vi "servo new.vi"() -> ()   [LabVIEW 2017]
panel:
  in  "Duty Cycle (%)":dbl=50.0
  out "error out":errorcluster
  in  "error in (no error)":errorcluster
  in  "Phase":dbl
  in  "Amplitude":dbl=1.0
  in  "Frequency":dbl=10.0
  in  "Reset Signal":bool
  in  "Offset":dbl
  out "Waveform Graph":dynamicdata(graph)
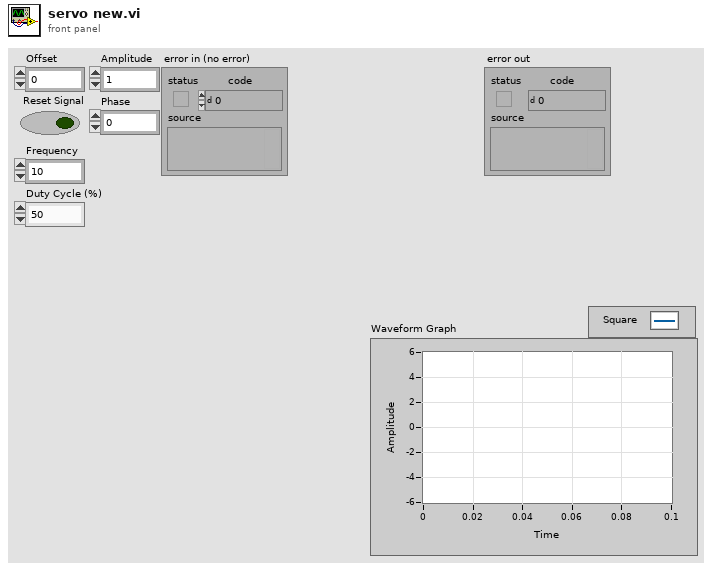
[diagram p1: front panel]
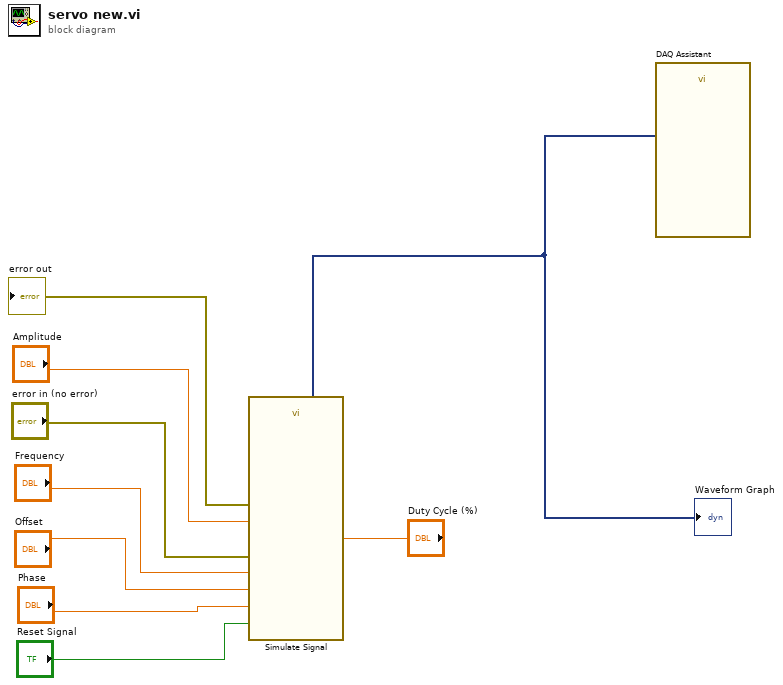
[diagram p0: block diagram]
diagram:
  n1 = call "Simulate Signal"("Offset"="Offset", "Duty Cycle (%)"="Duty Cycle (%)", "Reset Signal"="Reset Signal", "Frequency"="Frequency", "Amplitude"="Amplitude", "Phase"="Phase", "error in (no error)"="error in (no error)") -> ("Square"=w9:dynamicdata, "error out"=→"error out":errorcluster)  [unwired: 7 in]
  "Waveform Graph" <- w9
  n2 = call "DAQ Assistant"("data"=w9) -> ()  [unwired: 17 in, 2 out]
